vi "Axes XY Graph.vi"(9 "XYGraph Refnum":refnum<vi>, 11 "String":string) -> ()   [LabVIEW 2013]
doc: "Jean-Marc Simard \nExaprom inc. 2009"
panel:
  out "String[ ]":string[](array[string])
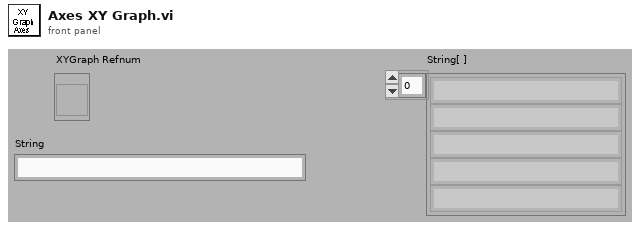
[diagram p1: front panel]
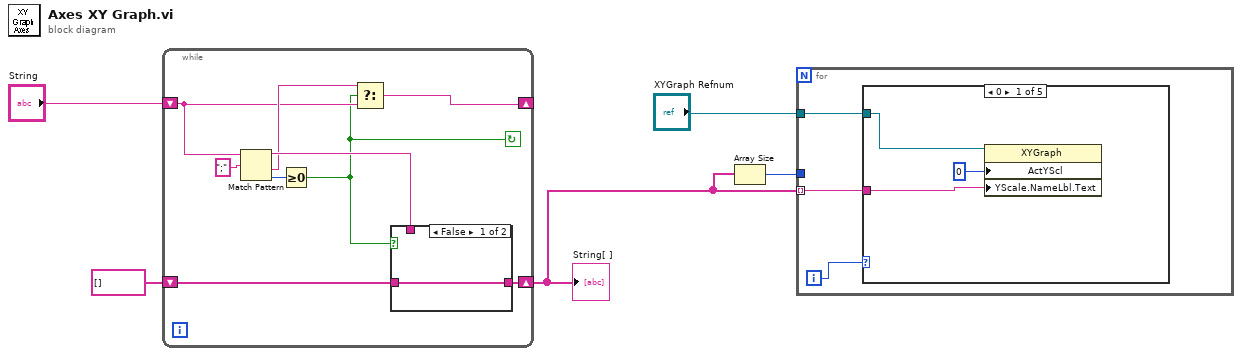
[diagram p0: block diagram]
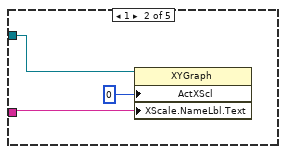
[diagram p2: hidden frame]
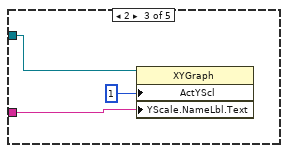
[diagram p3: hidden frame]
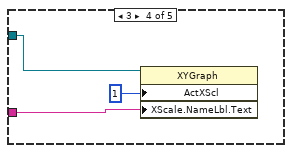
[diagram p4: hidden frame]
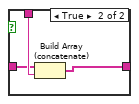
[diagram p6: hidden frame]
diagram:
  n1 = while {
    shift-right: [w12] -> _
    shift-left: "String" -> [w7]
    shift-right: [w9] -> w3
    shift-left: string[] [] ("String[ ]") -> [w10]
    stop <- w6 continue-if-true
    n2 = Match Pattern(string=w7, regular expression=";") -> (before substring=w11:string, after substring=w8:string, offset past match=w13:i32)  [unwired: 2 out]
    n3 = Greater Or Equal To 0?(x=w13) -> (x >= 0?=w6:bool)
    n4 = Select(t=w8, s=w6, f=w7) -> (s? t:f=w12:string)
    n5 = case shown="False" w6 {
      tunnel: w11 -> [_ w18]
      tunnel: w10 -> [w15 w17]
      tunnel: [w15 w16] -> w9
      frame False {
      }
      frame True {
        n6 = Build Array (concatenate)(w17, w18) -> (w16:string[])
      }
    }
  }
  "String[ ]" <- w3
  n7 = Array Size(array=w3) -> (size(s)=w2:i32)
  n8 = for {
    tunnel: "XYGraph Refnum" -> [w21]
    tunnel: w3 -> [w20] mode=indexing
    tunnel: w2 -> [_]
    i -> [w19]
    n9 = case shown="0" w19 {
      tunnel: w21 -> [w24 w25 w28 w31 _]
      tunnel: w20 -> [w22 w26 w29 w32 _]
      frame 0 {
        n10 = property class="XYGraph"(reference=w24, "ActYScl"=0 ("Active X Scale"), "YScale.NameLbl.Text"=w22) -> ()  [unwired: 1 in, 2 out]
      }
      frame 1 {
        n11 = property class="XYGraph"(reference=w25, "ActXScl"=0 ("Active X Scale"), "XScale.NameLbl.Text"=w26) -> ()  [unwired: 1 in, 2 out]
      }
      frame 2 {
        n12 = property class="XYGraph"(reference=w28, "ActYScl"=1 ("Active X Scale"), "YScale.NameLbl.Text"=w29) -> ()  [unwired: 1 in, 2 out]
      }
      frame 3 {
        n13 = property class="XYGraph"(reference=w31, "ActXScl"=1 ("Active X Scale"), "XScale.NameLbl.Text"=w32) -> ()  [unwired: 1 in, 2 out]
      }
      frame 4, Default {
      }
    }
  }
